vi "Select Color.vi"(8 "error in (no error)":errorcluster, 10 "Coords in":T1, 11 "ColorSelector in":refnum<class "ColorSelector.lvclass">) -> (0 "error out":errorcluster, 3 "ColorSelector (dup)":refnum<class "ColorSelector.lvclass">)   [LabVIEW 2015, in "ColorSelector.lvclass"]
doc: "Select Color determines the selected color from the Color Selector.\n<b> </b> <b> </b>\n©2017 Q Software Innovations, LLC (QSI)\nwritten by Quentin Alldredge\nproduced in LabVIEW 2015\n\nsupport@qsoftwareinnovations.com\nwww.qsoftwareinnovations.com\n\nAll rights reserved.\n\nRedistribution and use in source and binary forms, with or without modification, are permitted provided that the following conditions are met:\n\n * Redistributions of source code must retain the above copyright notice, this list of conditions and the following disclaimer.\n * Redistributions in binary form must reproduce the above copyright notice, this list of conditions and the following disclaimer in the documentation and/or other materials provided with the distribution.\n * Neither the name of Q Software Innovations, LLC. nor the names of its contributors may be used to endorse or promote products derived from this software without specific prior written permission.\n\nTHIS SOFTWARE IS PROVIDED BY THE COPYRIGHT HOLDERS AND CONTRIBUTORS \"AS IS\" AND ANY EXPRESS OR IMPLIED WARRANTIES, INCLUDING, BUT NOT LIMITED TO, THE IMPLIED WARRANTIES OF MERCHANTABILITY AND FITNESS FOR A PARTICULAR PURPOSE ARE DISCLAIMED. IN NO EVENT SHALL THE COPYRIGHT OWNER OR CONTRIBUTORS BE LIABLE FOR ANY DIRECT, INDIRECT, INCIDENTAL, SPECIAL, EXEMPLARY, OR CONSEQUENTIAL DAMAGES (INCLUDING, BUT NOT LIMITED TO, PROCUREMENT OF SUBSTITUTE GOODS OR SERVICES; LOSS OF USE, DATA, OR PROFITS; OR BUSINESS INTERRUPTION) HOWEVER CAUSED AND ON ANY THEORY OF LIABILITY, WHETHER IN CONTRACT, STRICT LIABILITY, OR TORT (INCLUDING NEGLIGENCE OR OTHERWISE) ARISING IN ANY WAY OUT OF THE USE OF THIS SOFTWARE, EVEN IF ADVISED OF THE POSSIBILITY OF SUCH DAMAGE."
uses:
  ColorSelector.lvclass
  <vilib>/Utility/miscctls.llb/LVPoint32TypeDef.ctl
  Write ColorGridCoords.vi
  Read ColorSelectPic.vi
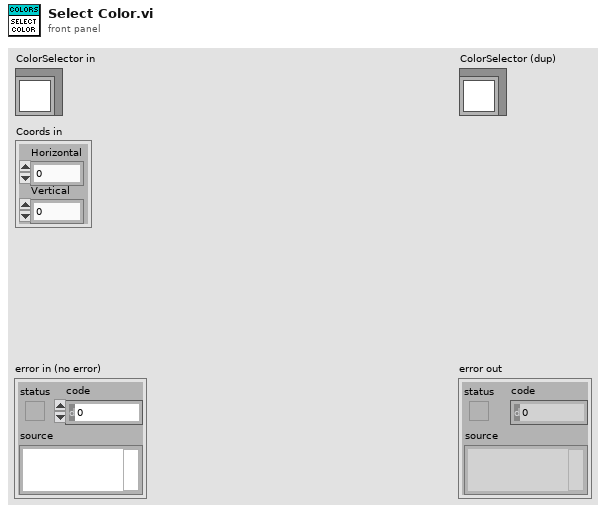
[diagram p1: front panel]
types:
  T1 = typedef "LVPoint32TypeDef.ctl" = cluster{"Horizontal":i32, "Vertical":i32}
  T2 = typedef "imagedata.ctl" = cluster{"image type":i32, "image depth":i32, "image":u8[], "mask":u8[], "colors":u32[], "Rectangle":cluster{"left":i16, "top":i16, "right":i16, "bottom":i16}}
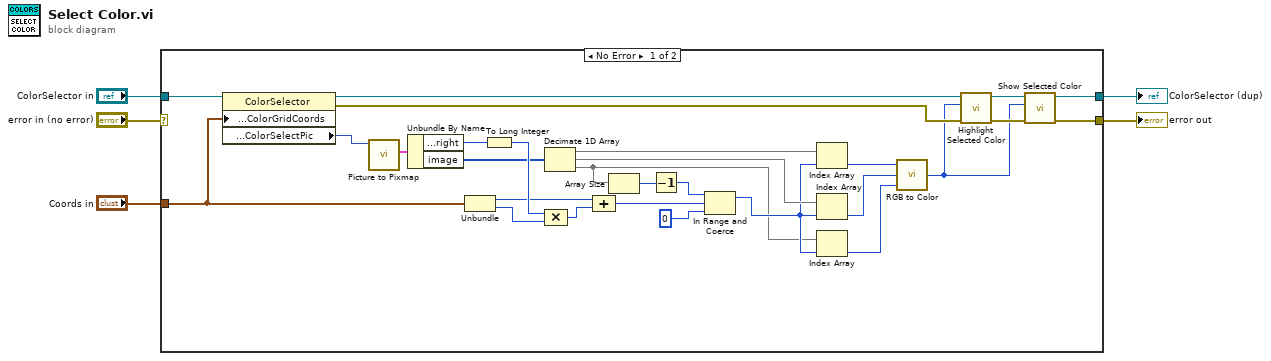
[diagram p0: block diagram]
diagram:
  n1 = case shown="No Error" "error in (no error)" {
    selector: "error in (no error)" -> [_ w35]
    tunnel: [w11 w35] -> w4
    tunnel: [w12 w34] -> w2
    tunnel: "ColorSelector in" -> [w8 w34]
    tunnel: "Coords in" -> [w7 _]
    frame No Error {
      n2 = property class="ColorSelector"(reference=w8, "State Data:Accessors:ColorGridCoords"=w7) -> (reference out=w10:refnum<class "ColorSelector.lvclass">, error out=w9:errorcluster, "State Data:Accessors:ColorSelectPic"=w20:picture)  [unwired: 1 in]
      n3 = call <vilib>:"Picture to Pixmap.vi"("picture"=w20) -> ("image data"=w33:T2)  [unwired: 9 in, 1 out]
      n4 = Unbundle By Name(w33) -> ("Rectangle.right"=w32:i16, "image"=w29:u8[])
      n5 = Unbundle(w7) -> ("Horizontal"=w16:i32, "Vertical"=w15:i32)
      n6 = To Long Integer(number=w32) -> (32bit integer=w31:i32)
      n7 = Decimate 1D Array(w29) -> (w28:u8[], w27:u8[], w19:u8[])
      n8 = Compound Arithmetic op=MULTIPLY(w31, w15) -> (w30:i32)
      n9 = Compound Arithmetic op=ADD(w16, w30) -> (w23:i32)
      n10 = Array Size(array=w19) -> (size(s)=w18:i32)
      n11 = Decrement(x=w18) -> (x-1=w17:i32)
      n12 = In Range and Coerce(upper limit=w17, x=w23, lower limit=0) -> (coerced(x)=w21:i32)  [unwired: 1 out]
      n13 = Index Array(array=w28, index=w21) -> (element=w26:u8)
      n14 = Index Array(array=w27, index=w21) -> (element=w25:u8)
      n15 = Index Array(array=w19, index=w21) -> (element=w24:u8)
      n16 = call <vilib>:"RGB to Color.vi"("B"=w24, "G"=w25, "R"=w26) -> ("Color"=w6:u32)
      n17 = call "Highlight Selected Color.vi"("error in (no error)"=w9, "Selected Color"=w6, "ColorSelector in"=w10) -> ("error out"=w13:errorcluster, "ColorSelector (dup)"=w14:refnum<class "ColorSelector.lvclass">)  [unwired: 7 in]
      n18 = call "Show Selected Color.vi"("error in (no error)"=w13, "Selected Color"=w6, "ColorSelector in"=w14) -> ("error out"=w11:errorcluster, "ColorSelector (dup)"=w12:refnum<class "ColorSelector.lvclass">)  [unwired: 7 in]
    }
    frame Error {
    }
  }
  "error out" <- w4
  "ColorSelector (dup)" <- w2
